vi "Read Data Queue.vi"(8 "error in (no error)":errorcluster, 11 "Analog Reader in":refnum<class "Analog Reader.lvclass">) -> (0 "error out":errorcluster, 2 "Data Queue":refnum<queue>, 3 "Analog Reader out":refnum<class "Analog Reader.lvclass">)   [LabVIEW 2024, in "DAQmx Actor.lvlib" / "Analog Reader.lvclass"]
uses:
  Analog Reader.lvclass
  Analog Reader.lvclass/Analog Reader.ctl
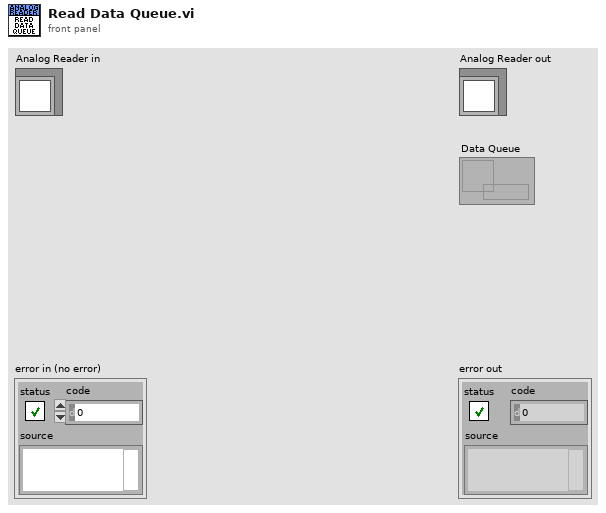
[diagram p1: front panel]
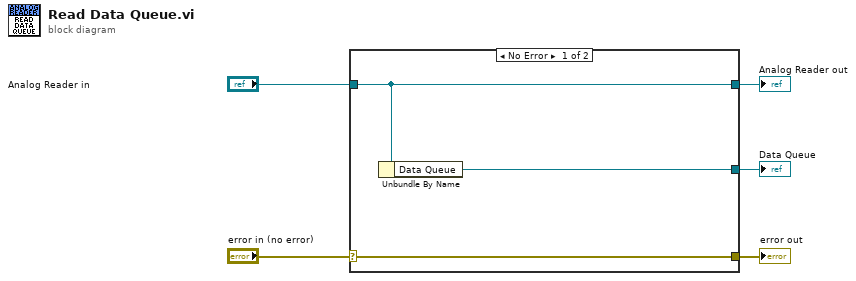
[diagram p0: block diagram]
diagram:
  n1 = case shown="No Error" "error in (no error)" {
    selector: "error in (no error)" -> [w8 w9]
    tunnel: [w8 w9] -> w4
    tunnel: [w7 w10] -> w2
    tunnel: "Analog Reader in" -> [w7 w10]
    tunnel: [w6 _] -> w1
    frame No Error {
      n2 = Unbundle By Name(w7) -> ("Data Queue"=w6:refnum<queue>)
    }
    frame Error {
    }
  }
  "error out" <- w4
  "Analog Reader out" <- w2
  "Data Queue" <- w1
